vi "Relative Seconds.vi"(9 "Relative Seconds in":dbl format="%_19f") -> (0 "Relative Seconds delta":dbl format="%_19f", 1 "Relative Seconds out":dbl format="%_19f", 7 "Dataflow Synch":variant)   [LabVIEW 2020, in "RTAF.lvlib"]
uses:
  RTAF.lvlib
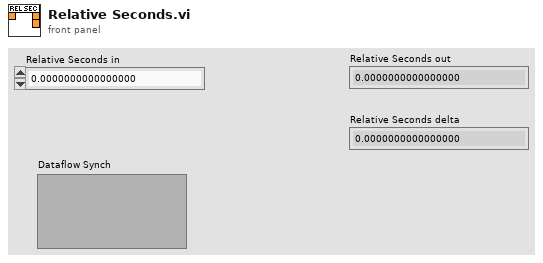
[diagram p1: front panel]
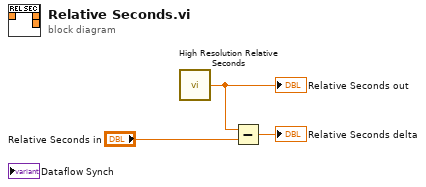
[diagram p0: block diagram]
diagram:
  n1 = call <vilib>:"High Resolution Relative Seconds.vi"() -> ("relative seconds"=w3:dbl)
  "Relative Seconds out" <- w3
  n2 = Subtract(x=w3, y="Relative Seconds in") -> (x-y=→"Relative Seconds delta":dbl)
